vi "Main-loop_backup.vi"() -> ()   [LabVIEW 2016]
uses:
  <vilib>/Platform/TimedLoop/XDataNode/timing_clust.ctl
  <vilib>/Platform/TimedLoop/XDataNode/nitl_modes.ctl
  <vilib>/Platform/TimedLoop/XDataNode/wakeup.ctl
  <vilib>/Utility/file.llb/Write Delimited Spreadsheet (DBL).vi
  <vilib>/Platform/TimedLoop/XDataNode/XDataNode.xnode
  <vilib>/Platform/TimedLoop/XDataNode/XDNodeRunTimeDep.lvlib
panel:
  out "error out 2":errorcluster
  out "Array":dbl[][](array[numeric])
  out "Region chart":cluster{dbl, dbl}(graph)
  out "error out":errorcluster
  in  "error in (no error)":errorcluster
  in  "stop main":bool
  out "Waveform Chart":cluster{dbl, dbl, dbl, dbl, dbl, dbl, dbl, dbl}(graph)
  in  "stop":bool
  out "Clock 2":i32
  out "Clock 1":i32
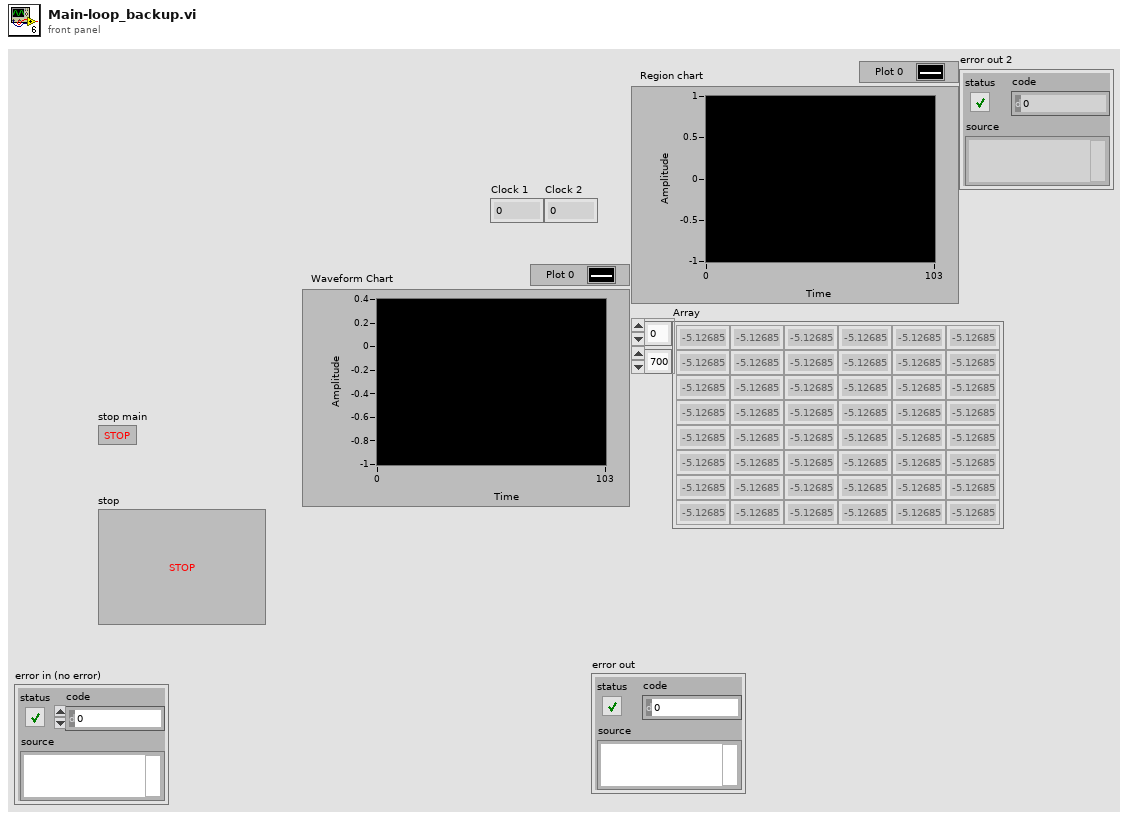
[diagram p1: front panel]
types:
  T1 = typedef "XDNodeRunTimeDep.lvlib/timing_clust.ctl" = cluster{"Expected End [f-1]":u64, "Actual End [f-1]":u64, "Finished Late? [f-1]":bool, "Expected End [i-1]":u64, "Actual End [i-1]":u64, "Finished Late? [i-1]":bool, "Expected Start [i]":u64, "Actual Start [i]":u64, "Expected Start [f]":u64, "Actual Start [f]":u64, "Source Name":string, "Structure Name":string, "Period":i64, "Deadline":i64, "Offset":i64, "Start":i64, "Priority":i32, "Timeout":i32, "Mode":T2, "Wakeup Reason":T3, "Error":errorcluster, "Source Type":string, "Secondary Source Type":string, "Global End Time":u64, "Global Start Time":u64, "Frame Duration":u64, "Iteration Duration":u64, "Assigned CPU":i32, "I/O Scan Engine Mode":u32}
  T2 = typedef "XDNodeRunTimeDep.lvlib/nitl_modes.ctl" = enum32{"No Change", "Process missed periods, maintain original phase", "Discard missed periods, maintain original phase", "Process missed periods, ignore original phase", "Discard missed periods, ignore original phase"}
  T3 = typedef "XDNodeRunTimeDep.lvlib/wakeup.ctl" = enum32{"Normal", "Aborted", "Asynchronous wakeup", "Timing source error", "Timed loop error", "Timeout"}
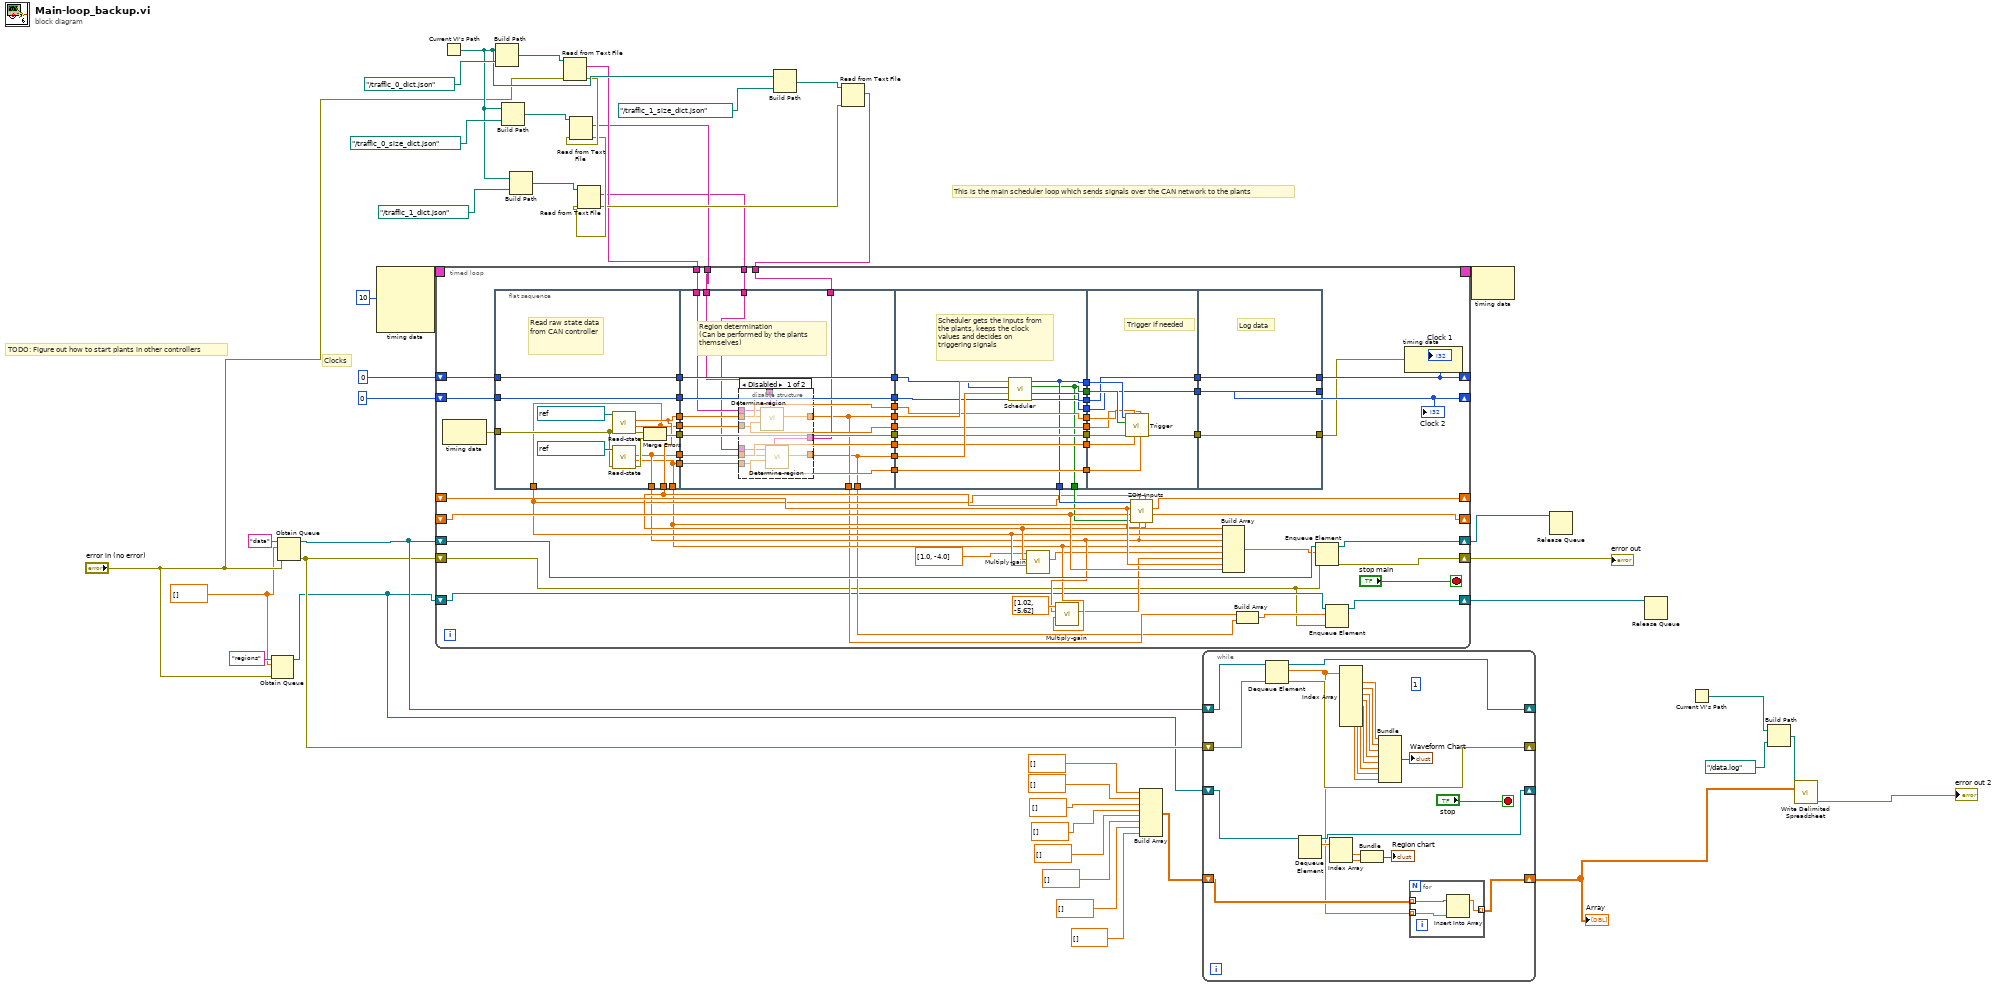
[diagram p0: block diagram]
diagram:
  w13 = dbl[] []
  # "Clocks"
  # "TODO: Figure out how to start plants in other controllers"
  # "This is the main scheduler loop which sends signals over the CAN network to the plants"
  n1 = Obtain Queue(name (unnamed)="regions", element data type=w13, error in (no error)="error in (no error)") -> (queue out=w12:refnum<queue>)  [unwired: 2 in, 2 out]
  n2 = Obtain Queue(name (unnamed)="data", element data type=w13, error in (no error)="error in (no error)") -> (queue out=w39:refnum<queue>, error out=w38:errorcluster)  [unwired: 2 in, 1 out]
  n3 = node-c288(i64 10 ("Period")) -> (w45:T1)  [unwired: 3 in]
  n4 = Current VI's Path() -> (path=w27:path)
  n5 = Build Path(base path=w27, name or relative path=path "../traffic_0_dict.json") -> (appended path=w35:path)
  n6 = Build Path(base path=w27, name or relative path=path "../traffic_0_size_dict.json") -> (appended path=w32:path)
  n7 = Build Path(base path=w27, name or relative path=path "../traffic_1_dict.json") -> (appended path=w31:path)
  n8 = Read from Text File(file (use dialog)=w35, error in="error in (no error)") -> (text=w19:string, error out=w22:errorcluster)  [unwired: 2 in, 2 out]
  n9 = Read from Text File(file (use dialog)=w32, error in=w22) -> (text=w18:string, error out=w21:errorcluster)  [unwired: 2 in, 2 out]
  n10 = Read from Text File(file (use dialog)=w31, error in=w21) -> (text=w17:string, error out=w20:errorcluster)  [unwired: 2 in, 2 out]
  n11 = Build Path(base path=w27, name or relative path=path "../traffic_1_size_dict.json") -> (appended path=w28:path)
  n12 = Read from Text File(file (use dialog)=w28, error in=w20) -> (text=w16:string)  [unwired: 2 in, 3 out]
  n13 = timed-loop {
    timing: w45 -> [_]
    timing-out: [_] -> w44
    shift-right: [w93] -> _
    shift-left: 0 -> [w107]
    shift-right: [w90] -> _
    shift-left: 0 -> [w108]
    shift-right: [w66] -> w26
    shift-left: w38 -> [w46]
    shift-right: [w67] -> w7
    shift-left: w39 -> [w69]
    shift-right: [w73] -> _
    shift-left: _ -> [w71]
    shift-right: [w72] -> _
    shift-left: _ -> [w70]
    tunnel: w19 -> [w63]
    tunnel: w18 -> [w62]
    tunnel: w17 -> [w61]
    tunnel: w16 -> [w60]
    shift-right: [w48] -> w6
    shift-left: w12 -> [w47]
    stop <- "stop main" stop-if-true
    n14 = node-c288() -> (w104:errorcluster)  [unwired: 1 in]
    n15 = flat-sequence {
      tunnel: w107 -> [w119]
      tunnel: w108 -> [w120]
      tunnel: [w120] -> w106
      tunnel: [w119] -> w105
      tunnel: w104 -> [w116]
      tunnel: [w110] -> w103
      tunnel: [w109] -> w102
      tunnel: [w111] -> w101
      tunnel: [w112] -> w100
      tunnel: [w113] -> w87
      tunnel: [w112] -> w59
      tunnel: [w111] -> w58
      tunnel: [w110] -> w55
      tunnel: [w109] -> w54
      tunnel: w106 -> [w132]
      tunnel: w105 -> [w133]
      tunnel: w103 -> [w128]
      tunnel: w102 -> [w127]
      tunnel: w101 -> [w129]
      tunnel: w100 -> [w130]
      tunnel: [w122] -> w99
      tunnel: [w121] -> w98
      tunnel: [w133] -> w97
      tunnel: [w132] -> w96
      tunnel: [w131] -> w88
      tunnel: w87 -> [w131]
      tunnel: [w130] -> w84
      tunnel: [w129] -> w82
      tunnel: [w128] -> w81
      tunnel: [w127] -> w78
      tunnel: w63 -> [w126]
      tunnel: w62 -> [w125]
      tunnel: w61 -> [w124]
      tunnel: w60 -> [w123]
      tunnel: [w122] -> w51
      tunnel: [w121] -> w50
      tunnel: w99 -> [w156]
      tunnel: w98 -> [w155]
      tunnel: w97 -> [w154]
      tunnel: w96 -> [w153]
      tunnel: [w145] -> w95
      tunnel: [w144] -> w94
      tunnel: [w152] -> w92
      tunnel: [w151] -> w91
      tunnel: [w150] -> w89
      tunnel: w88 -> [w150]
      tunnel: [w149] -> w85
      tunnel: w84 -> [w149]
      tunnel: [w148] -> w83
      tunnel: w82 -> [w148]
      tunnel: w81 -> [w147]
      tunnel: [w147] -> w80
      tunnel: [w146] -> w79
      tunnel: w78 -> [w146]
      tunnel: [w145] -> w74
      tunnel: [w144] -> w64
      tunnel: w95 -> [w166]
      tunnel: w94 -> [w165]
      tunnel: w92 -> [w164]
      tunnel: w91 -> [w163]
      tunnel: w89 -> [w162]
      tunnel: w85 -> [w160]
      tunnel: w83 -> [w159]
      tunnel: w80 -> [w158]
      tunnel: w79 -> [w157]
      tunnel: [w164] -> w77
      tunnel: [w163] -> w76
      tunnel: [w161] -> w75
      tunnel: [w167] -> w86
      tunnel: [w168] -> w90
      tunnel: [w169] -> w93
      tunnel: w77 -> [w169]
      tunnel: w76 -> [w168]
      tunnel: w75 -> [w167]
      frame #0 {
        # "Read raw state data from CAN controller"
        n16 = call "Read-state.vi"("error in (no error)"=w116, "XNET Session"=refnum<k21> "Plant1_state") -> ("error out"=w114:errorcluster, "X2"=w111:dbl, "X1"=w112:dbl)  [unwired: 7 in]
        n17 = call "Read-state.vi"("error in (no error)"=w116, "XNET Session"=refnum<k21> "Plant2_state") -> ("error out"=w115:errorcluster, "X2"=w109:dbl, "X1"=w110:dbl)  [unwired: 7 in]
        n18 = Merge Errors(w114, w115) -> (w113:errorcluster)
      }
      frame #1 {
        # "Region determination \n(Can be performed by the plants\nthemselves)"
        n19 = disable-structure shown="Disabled" {
          disable-tunnel: w130 -> [w143 _]
          disable-tunnel: w129 -> [w142 _]
          disable-tunnel: w128 -> [w141 _]
          disable-tunnel: w127 -> [w140 _]
          disable-tunnel: w126 -> [w139 _]
          disable-tunnel: w125 -> [w138 _]
          disable-tunnel: w124 -> [w137 _]
          disable-tunnel: w123 -> [w136 _]
          disable-tunnel: [w135 _] -> w122
          disable-tunnel: [w134 _] -> w121
          frame Disabled {
            n20 = call "Determine-region.vi"("JSON information string"=w138, "X2"=w142, "X1"=w143, "JSON string for Q matrices"=w139) -> ("Region"=w135:dbl)  [unwired: 7 in]
            n21 = call "Determine-region.vi"("JSON information string"=w136, "X2"=w140, "X1"=w141, "JSON string for Q matrices"=w137) -> ("Region"=w134:dbl)  [unwired: 7 in]
          }
          frame Enabled {
          }
        }
      }
      frame #2 {
        # "Scheduler gets the inputs from the plants, keeps the clock values and decides on triggering signals"
        n22 = call "Scheduler.vi"("Clock, plant 2"=w153, "Region, plant 2"=w155, "Clock, plant 1"=w154, "Region, plant 1"=w156) -> ("Clock 2"=w151:i32, "Clock 1"=w152:i32, "Trigger?"=w144:bool, "Plant to trigg"=w145:enum16{"Plant 1", "Plant 2"})  [unwired: 4 in]
      }
      frame #3 {
        # "Trigger if needed"
        n23 = call "Trigger.vi"("Plant 2 X2"=w157, "Plant 1 X2"=w159, "Plant 2 X1"=w158, "Plant 1 X1"=w160, "error in (no error)"=w162, "Trigger"=w165, "Plant to trigg"=w166) -> ("error out"=w161:errorcluster)  [unwired: 4 in]
      }
      frame #4 {
        # "Log data"
      }
    }
    n24 = call "Multiply-gain.vi"("X2"=w58, "X1"=w59, "Gain (K)"=dbl[] [1.0, -4.0]) -> ("Kx"=w53:dbl)  [unwired: 8 in]
    n25 = call "Multiply-gain.vi"("X2"=w54, "X1"=w55, "Gain (K)"=dbl[] [1.02, -5.62]) -> ("Kx"=w52:dbl)  [unwired: 8 in]
    n26 = call "ZOH-Inputs.vi"("Plant 2 X2"=w54, "Plant 1 X2"=w58, "Plant 2 X1"=w55, "Plant 1 X1"=w59, "Trigger"=w64, "Plant 2 KX Hat"=w70, "Plant 1 KX hat"=w71, "Plant to trigg"=w74) -> ("Plant 2 KX Hat"=w72:dbl, "Plant 1 KX hat"=w73:dbl)  [unwired: 2 in]
    n27 = Build Array(w59, w58, w55, w54, w53, w52, w71, w70) -> (w68:dbl[])
    n28 = Build Array(w51, w50) -> (w49:dbl[])
    n29 = Enqueue Element(queue=w69, element=w68, error in (no error)=w46) -> (queue out=w67:refnum<queue>, error out=w66:errorcluster)  [unwired: 1 in, 1 out]
    n30 = Enqueue Element(queue=w47, element=w49, error in (no error)=w46) -> (queue out=w48:refnum<queue>)  [unwired: 1 in, 2 out]
    n31 = node-c288(w86) -> ()  [unwired: 1 out]
    "Clock 1" <- w93
    "Clock 2" <- w90
  }
  "error out" <- w26
  n32 = Build Array(dbl[] [], dbl[] [], dbl[] [], dbl[] [], dbl[] [], dbl[] [] ("element"), dbl[] [] ("element"), dbl[] [] ("element")) -> (w8:dbl[][])
  n33 = while {
    shift-right: [w195] -> _
    shift-left: w39 -> [w196]
    shift-right: [w194] -> _
    shift-left: w38 -> [w197]
    shift-right: [w191] -> _
    shift-left: w12 -> [w192]
    shift-right: [w175] -> w5
    shift-left: w8 -> [w177]
    stop <- "stop" stop-if-true
    (unwired) 1 ("dimension size")
    n34 = Dequeue Element(queue=w196, error in (no error)=w197) -> (queue out=w195:refnum<queue>, element=w176:dbl[], error out=w194:errorcluster)  [unwired: 1 in, 1 out]
    n35 = Dequeue Element(queue=w192) -> (queue out=w191:refnum<queue>, element=w190:dbl[])  [unwired: 2 in, 2 out]
    n36 = Index Array(array=w190) -> (element #1=w189:dbl, element #2=w188:dbl)  [unwired: 2 in]
    n37 = Index Array(array=w176) -> (element #1=w178:dbl, element #2=w185:dbl, element #3=w184:dbl, element #4=w183:dbl, element #5=w182:dbl, element #6=w181:dbl, element #7=w180:dbl, element #8=w179:dbl)  [unwired: 8 in]
    n38 = Bundle(w189, w188) -> (→"Region chart":cluster{dbl, dbl})  [unwired: 1 in]
    n39 = Bundle(w178, w185, w184, w183, w182, w181, w180, w179) -> (→"Waveform Chart":cluster{dbl, dbl, dbl, dbl, dbl, dbl, dbl, dbl})  [unwired: 1 in]
    n40 = for {
      tunnel: w177 -> [w200] mode=indexing
      tunnel: w176 -> [w199] mode=indexing
      tunnel: [w198] -> w175 mode=indexing
      n41 = Insert Into Array(array=w200, new element=w199) -> (w198:dbl[])  [unwired: 1 in]
    }
  }
  "Array" <- w5
  n42 = node-c288(w44) -> ()  [unwired: 1 out]
  n43 = Release Queue(queue=w7) -> ()  [unwired: 2 in, 3 out]
  n44 = Release Queue(queue=w6) -> ()  [unwired: 2 in, 3 out]
  n45 = Current VI's Path() -> (path=w3:path)
  n46 = Build Path(base path=w3, name or relative path=path "../data.log" ("file path (dialog if empty)")) -> (appended path=w1:path)
  n47 = call-poly <vilib>:"Write Delimited Spreadsheet.vi"("file path (dialog if empty)"=w1, "2D data"=w5) -> ("error out"=→"error out 2":errorcluster)  [unwired: 12 in, 1 out]
